vi "TDMS - File Viewer - KTMod1.vi"(4 "error in (no error)":errorcluster, 7 "file path":path) -> (0 "error out":errorcluster, 3 "file path out":path)   [LabVIEW 2019]
doc: "Developed by Kevin Thompson\nkevin@thompsonengineering.net\n\nCopyright 2020\nThompson Engineering, LLC\n<B>Copyright:</B> (c) 2017 National Instruments. All rights reserved.\n\nOpens the .tdms file specified in the <B>file path</B> input and presents the file data in the TDMS File Viewer dialog box."
uses:
  Instance           1 26Saved   TDMS - File Viewer .vi
  <vilib>/Utility/tdmsutil.llb/fileViewerConfigData.ctl
  <vilib>/Utility/tdmsutil.llb/TDMSFileViewerLocalizedText.vi
  <vilib>/Utility/error.llb/DialogType.ctl
  <vilib>/event_ctls.llb/sizeaction.ctl
  <vilib>/event_ctls.llb/panelstate.ctl
panel:
  out "LastXScaleFormat":u8
  out "TotalCount":u64
  out "Temp Configuration":T1
  in  "LastTopLeftValue":u64
  out "Resize?":bool
  in  "Help":bool
  in  "Status":string
  in  "Quit":bool
  in  "Settings...":bool
  in  "Properties / Values / Graph":T2(tab)
  in  "Properties":i32(listbox)
  in  "Go To":bool
  in  "Scrollbar":u64(c297)
  in  "Raw data values":i32(listbox)
  out "Waveform Graph":waveform(dbl)[](graph)
  in  "File contents":string(tree)
  # "Right Click for File Dialog"
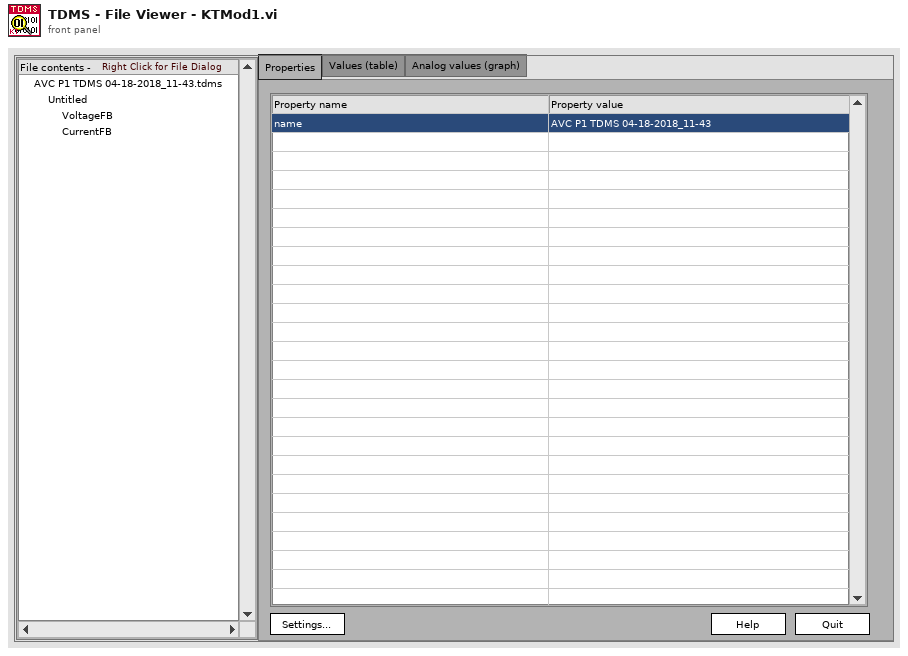
[diagram p1: front panel]
types:
  T1 = typedef "fileViewerConfigData.ctl" = cluster{"Show all (table)":bool, "Show all (graph)":bool, "limit (table)":u64, "limit (graph)":u64, "no show":bool, "start (table)":u64, "start (graph)":u64}
  T2 = enum32{"Properties", "Values (table)", "Analog values (graph)"}
  T3 = enum16{"open", "open or create", "create or replace", "create", "open (read-only)"}
  T4 = cluster{"Tree":refnum<vi>, "Tab Control":refnum<vi>, "property list":refnum<vi>, "raw data list":refnum<vi>, "Waveform Graph":refnum<vi>, "Ok":refnum<vi>, "Ok 2":refnum<vi>, "Ok 3":refnum<vi>, "Ok 4":refnum<vi>, "Scrollbar":refnum<vi>, "Ok 5":refnum<vi>, "TopLeftValue":refnum<vi>, "TotalCount":refnum<vi>}
  T5 = typedef "panelstate.ctl" = enum32{"Standard", "Minimized", "Maximized"}
  T6 = typedef "sizeaction.ctl" = enum32{"Minimized", "Maximized", "Resized"}
  T7 = cluster{"Shift":bool, "Ctrl":bool, "Alt":bool, "Cmd":bool, "Opt":bool}
  T8 = typedef "LVRectTypeDef.ctl" = cluster{"Left":i16, "Top":i16, "Right":i16, "Bottom":i16}
  T9 = typedef "LVRowAndColumnUnsignedTypeDef.ctl" = cluster{"Row":u32, "Column":u32}
  T10 = typedef "DialogType.ctl" = u16
  T11 = typedef "eventvkey.ctl" = enum16{"ASCII", "Enter", "Return", "Shift", "Ctrl", "Alt", "Cmd", "Opt", "Caps", "NumLock", "Clear", "Break", "Up", "Down", "Left", "Right", "Insert", "Delete", "Home", "End", "PageUp", "PageDown", "Escape", "Help", "Pause", "ScrollLock", "F1", "F2", "F3", "F4", "F5", "F6", "F7", "F8", "F9", "F10", "F11", "F12", "F13", "F14", "F15", "F16", "F17", "F18", "F19", "F20", "F21", "F22", "F23", "F24", "Play", "VolumeUp", "VolumeDown", "Mute", "Two Byte Char"}
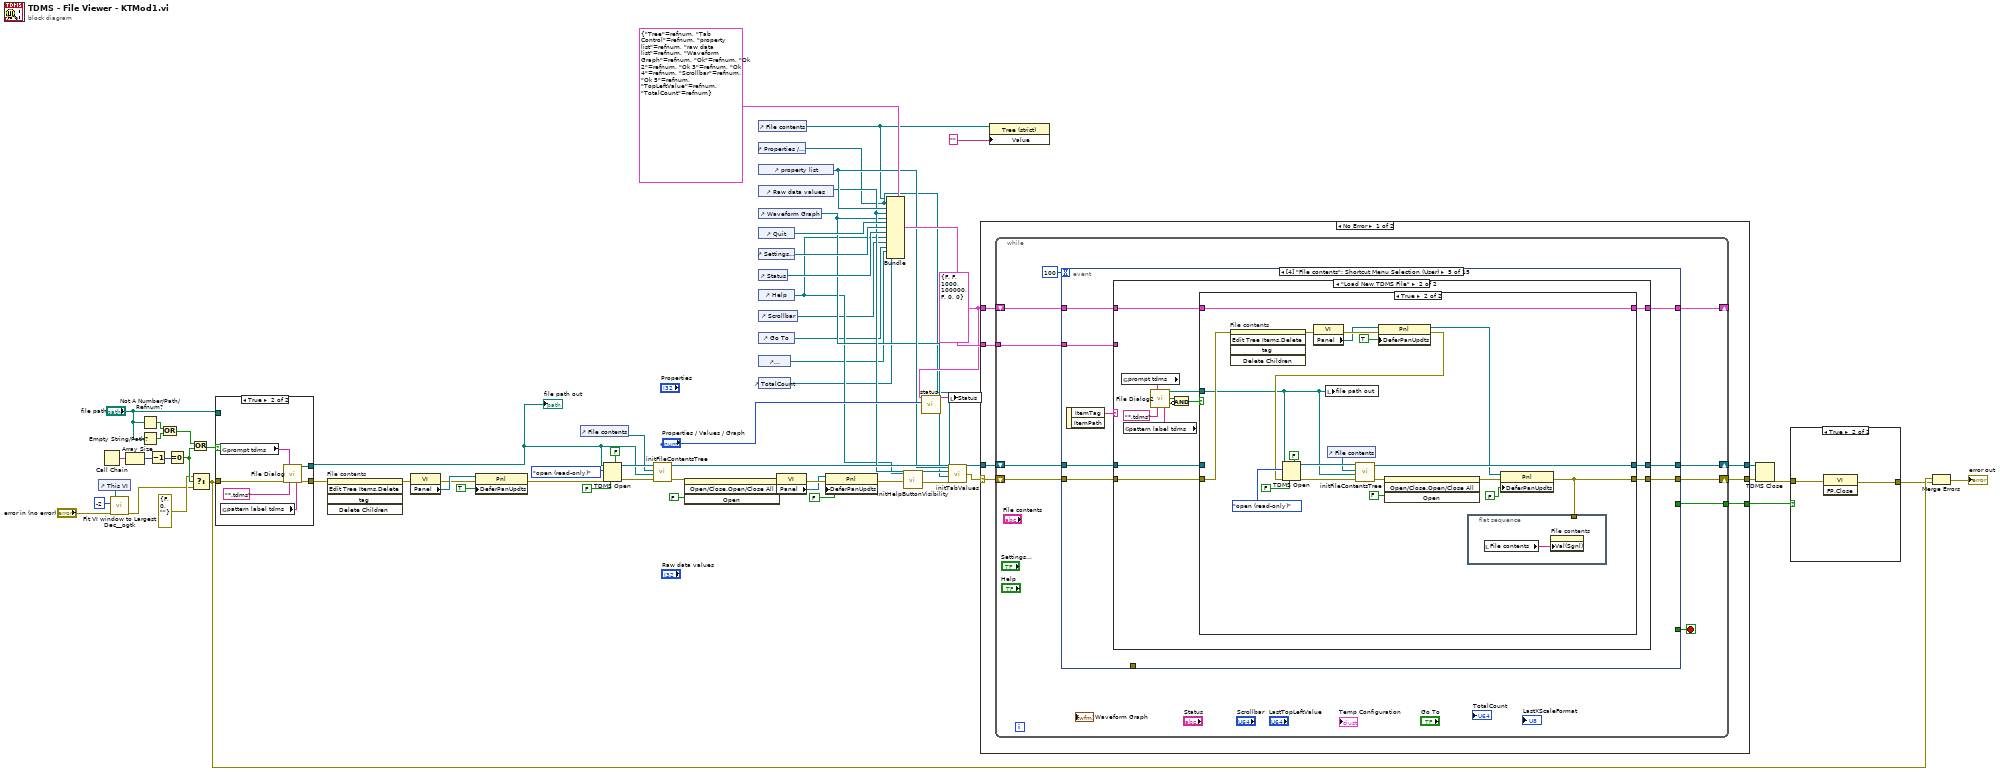
[diagram p0: block diagram]
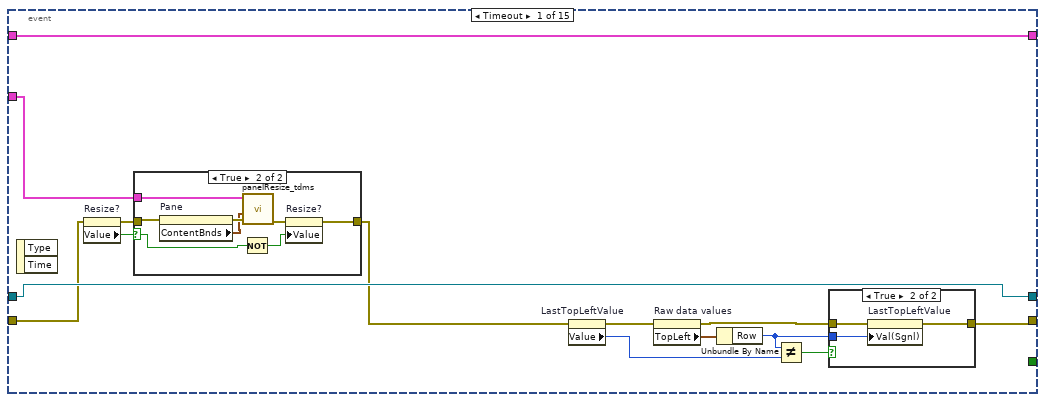
[diagram p3: hidden frame]
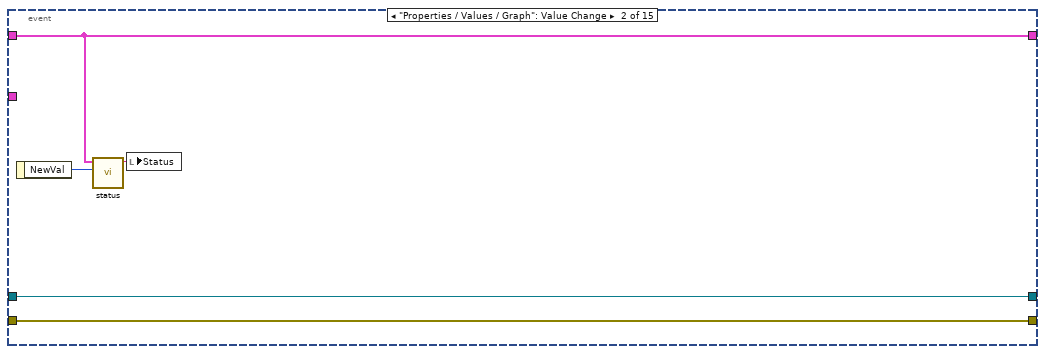
[diagram p6: hidden frame]
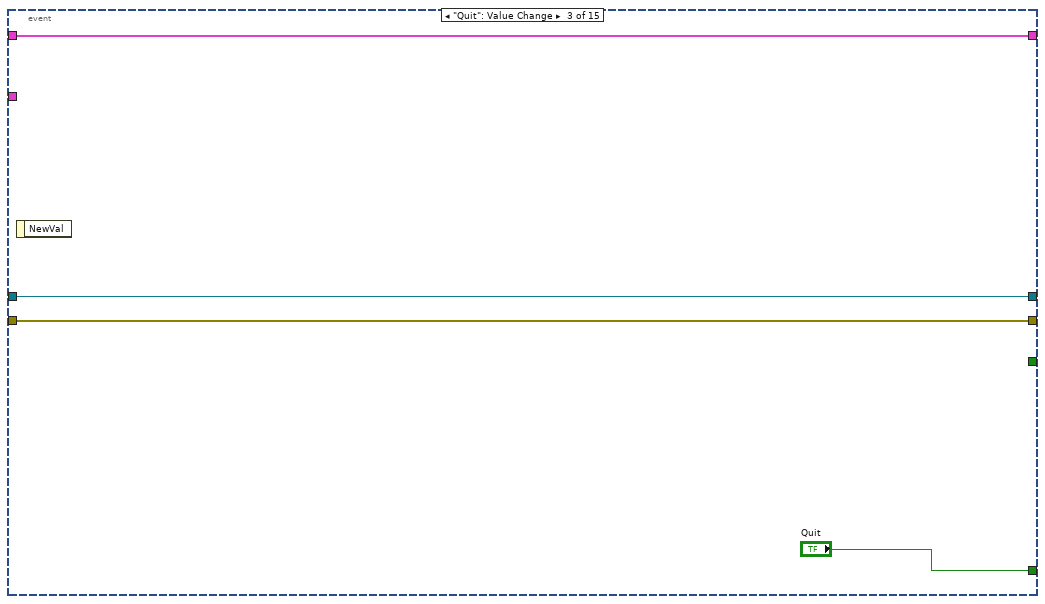
[diagram p7: hidden frame]
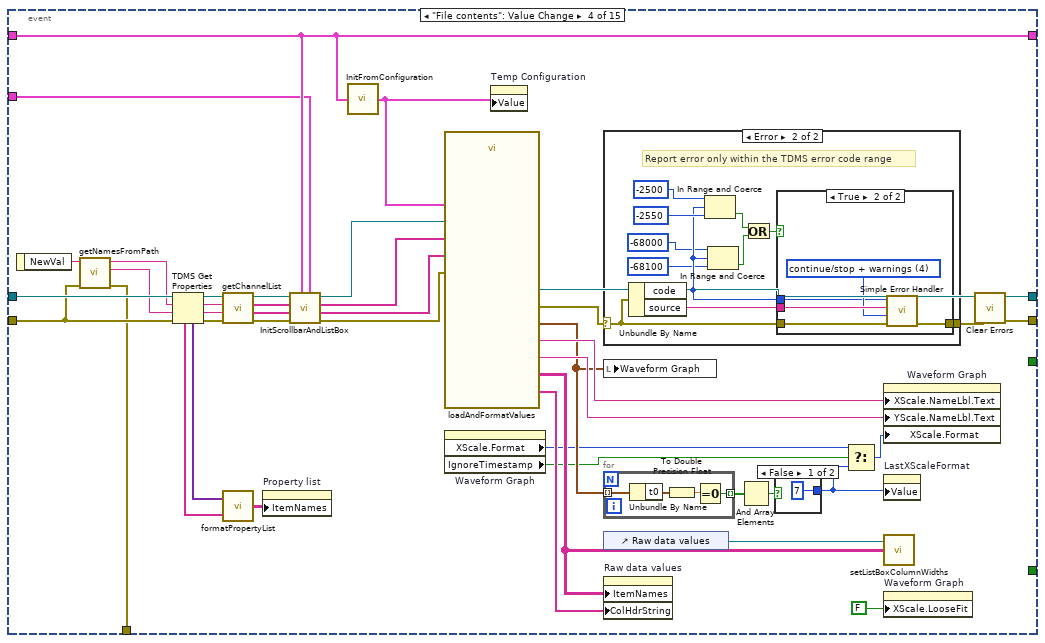
[diagram p8: hidden frame]
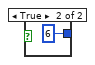
[diagram p9: hidden frame]
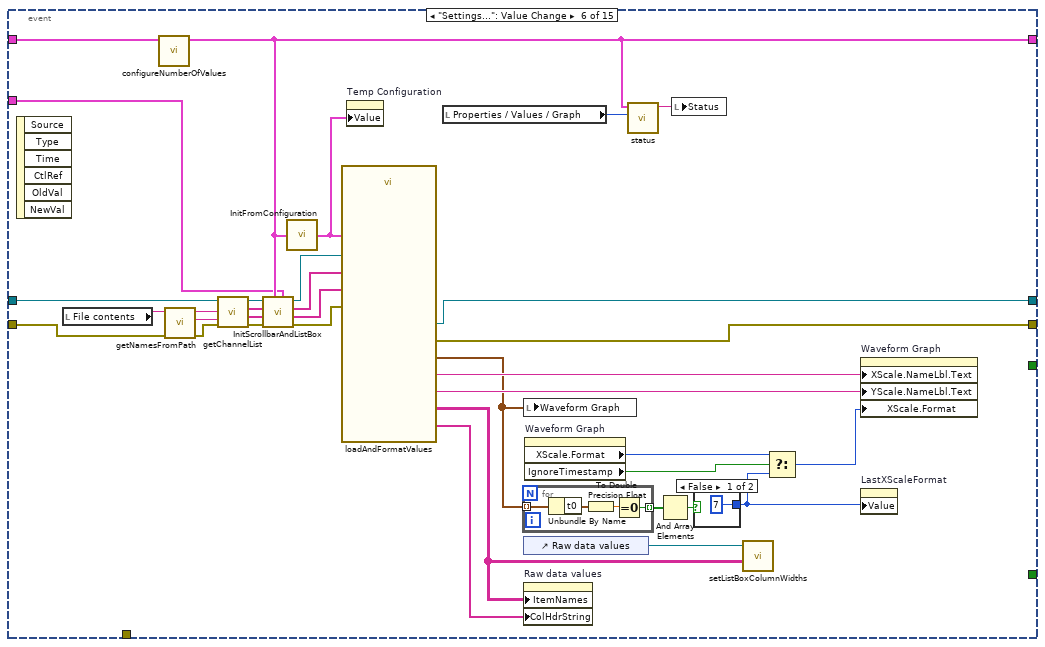
[diagram p14: hidden frame]
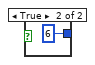
[diagram p15: hidden frame]
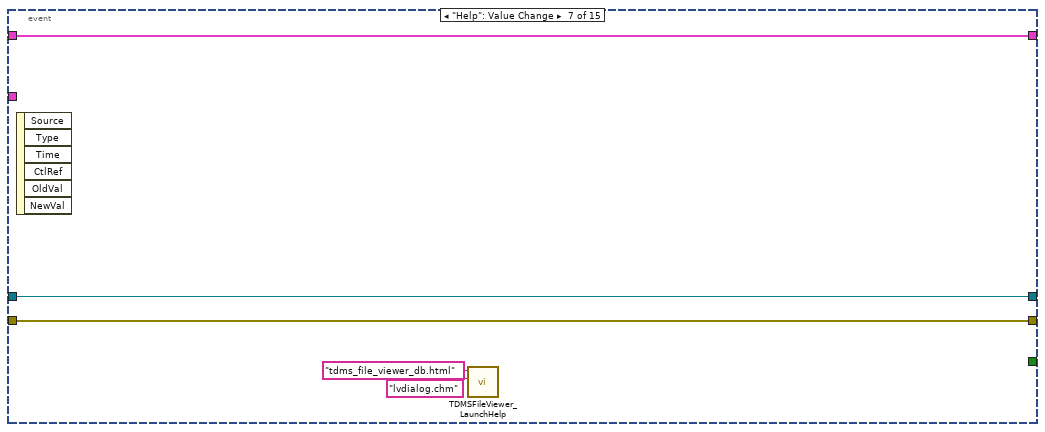
[diagram p16: hidden frame]
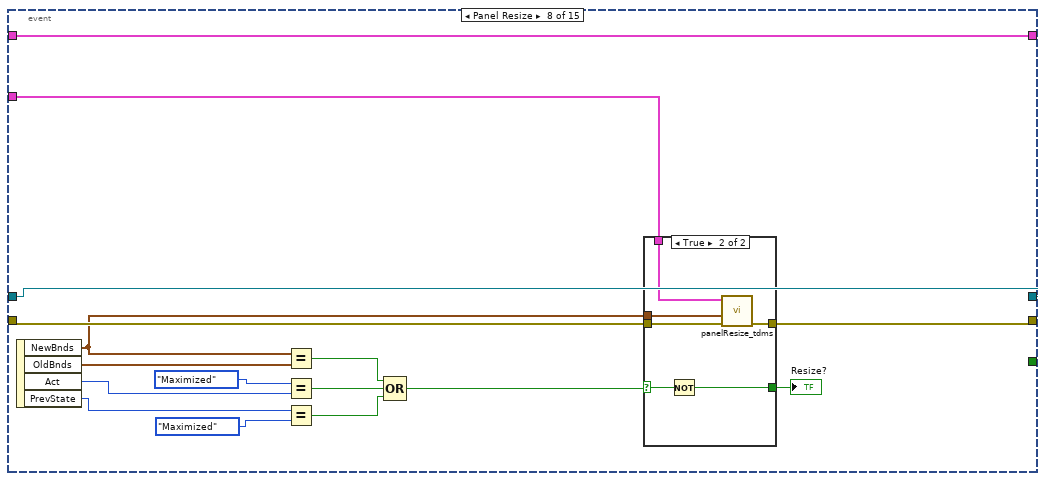
[diagram p17: hidden frame]
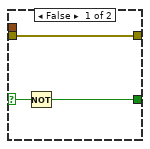
[diagram p18: hidden frame]
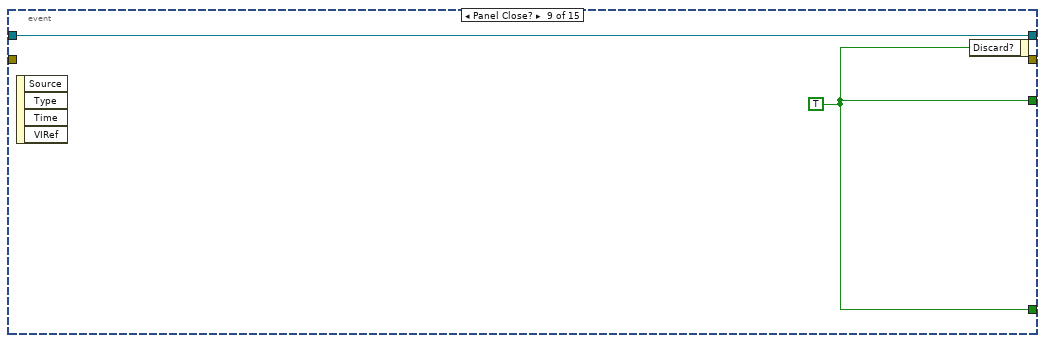
[diagram p19: hidden frame]
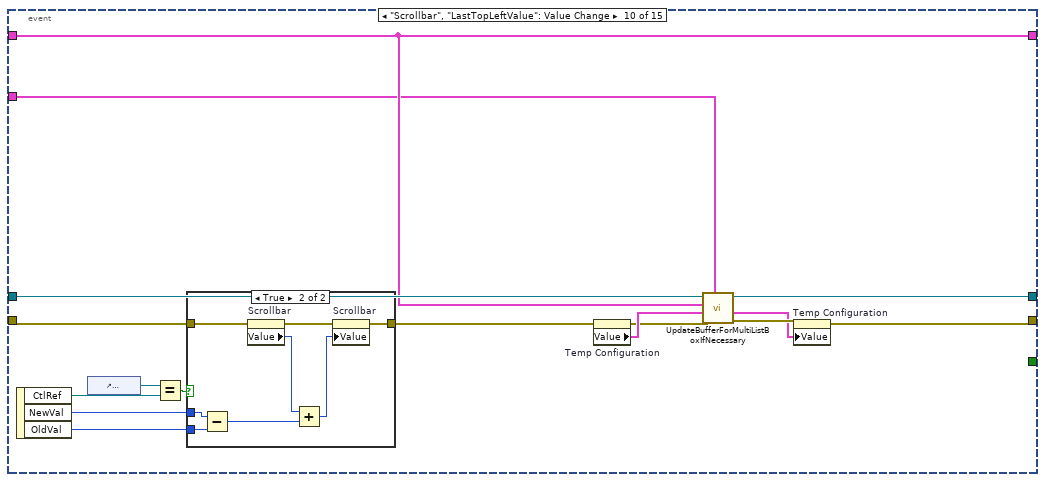
[diagram p20: hidden frame]
diagram:
  w29 = T1 {"Show all (table)"=FALSE, "Show all (graph)"=FALSE, "limit (table)"=1000, "limit (graph)"=100000, "no show"=FALSE, "start (table)"=0, "start (graph)"=0} ("TDMS File Viewer Configuration")
  n1 = control-ref of="This VI"() -> (w4:refnum<vi>)
  n2 = Call Chain() -> (call chain=w44:string[])
  n3 = call <userlib>:"Fit VI window to Largest Dec__ogtk.vi"("error in (no error)"="error in (no error)", "border spacing (2 px)"=-2, "VI Ref (calling VI)"=w4) -> ("error out"=w1:errorcluster)  [unwired: 3 in, 1 out]
  n4 = Array Size(array=w44) -> (size(s)=w42:i32)
  n5 = Not A Number/Path/Refnum?(number/path/refnum="file path") -> (NaN/Path/Refnum?=w46:bool)
  n6 = Empty String/Path?(string/path="file path") -> (empty?=w45:bool)
  n7 = Decrement(x=w42) -> (x-1=w41:i32)
  n8 = Or(x=w46, y=w45) -> (x .or. y?=w43:bool)
  n9 = Equal To 0?(x=w41) -> (x = 0?=w27:bool)
  n10 = Or(x=w43, y=w27) -> (x .or. y?=w40:bool)
  n11 = Select(t=errorcluster {"status"=FALSE, "code"=0, "source"=""}, s=w27, f=w1) -> (s? t:f=w11:errorcluster)
  n12 = case shown="True" w40 {
    tunnel: [w65 w71] -> w33
    tunnel: "file path" -> [w65 _]
    tunnel: [w64 w69] -> w32
    tunnel: w11 -> [w64 w68]
    frame False {
    }
    frame True {
      n13 = global read "TDMSFileViewerLocalizedText.vi" "prompt tdms"() -> (w67:string)
      n14 = global read "TDMSFileViewerLocalizedText.vi" "pattern label tdms"() -> (w66:string)
      n15 = call "File Dialog"("prompt"=w67, "error in"=w68, "pattern (all files)"="*.tdms", "pattern label"=w66) -> ("selected path"=w71:path, "error out"=w69:errorcluster)  [unwired: 3 in, 7 out]
    }
  }
  "file path out" <- w33
  n16 = invoke on="File contents" class="Tree (strict)" method="Edit Tree Items.Delete"(error in=w32) -> (error out=w54:errorcluster)  [unwired: 4 in, 4 out]
  n17 = property class="VI"(error in=w54) -> (error out=w55:errorcluster, "Panel"=w56:refnum<vi>)  [unwired: 1 in, 1 out]
  n18 = property class="Pnl"(reference=w56, error in=w55, "DeferPanUpdts"=TRUE ("Defer Panel Updates")) -> (error out=w58:errorcluster)  [unwired: 1 out]
  n19 = control-ref of="File contents"() -> (w34:refnum<vi>)
  n20 = TDMS Open(5:FALSE ("create index file? (T)"), 6:FALSE ("disable buffering (T)"), 8:w58, 10:T3."open (read-only)" ("operation"), 11:w33) -> (0:w63:errorcluster, 3:w62:refnum<k34>)  [unwired: 2 in]
  n21 = call <vilib>:"initFileContentsTree.vi"("error in (no error)"=w63, "file path"=w33, "Tree Refnum"=w34, "tdms file"=w62) -> ("error out"=w50:errorcluster, "tdms file out"=w61:refnum<k34>)  [unwired: 2 out]
  n22 = invoke on="File contents" class="Tree (strict)" method="Open/Close.Open/Close All"(error in=w50, "Open"=FALSE ("Open?")) -> (error out=w49:errorcluster)  [unwired: 2 in, 3 out]
  n23 = control-ref of="File contents"() -> (w17:refnum<vi>)
  n24 = control-ref of="property list"() -> (w21:refnum<vi>)
  n25 = control-ref of="Raw data values"() -> (w20:refnum<vi>)
  n26 = control-ref of="Waveform Graph"() -> (w19:refnum<vi>)
  n27 = control-ref of="Quit"() -> (w38:refnum<vi>)
  n28 = control-ref of="Settings..."() -> (w36:refnum<vi>)
  n29 = control-ref of="Status"() -> (w31:refnum<vi>)
  n30 = control-ref of="Help"() -> (w13:refnum<vi>)
  n31 = control-ref of="Scrollbar"() -> (w10:refnum<vi>)
  n32 = control-ref of="Go To"() -> (w9:refnum<vi>)
  n33 = control-ref of="LastTopLeftValue"() -> (w8:refnum<vi>)
  n34 = control-ref of="TotalCount"() -> (w7:refnum<vi>)
  n35 = control-ref of="Properties / Values / Graph"() -> (w18:refnum<vi>)
  n36 = property class="VI"(error in=w49) -> (error out=w52:errorcluster, "Panel"=w51:refnum<vi>)  [unwired: 1 in, 1 out]
  n37 = property class="Pnl"(reference=w51, error in=w52, "DeferPanUpdts"=FALSE ("Defer Panel Updates")) -> (error out=w15:errorcluster)  [unwired: 1 out]
  n38 = Bundle(cluster=T4 {"Tree"=refnum, "Tab Control"=refnum, "property list"=refnum, "raw data list"=refnum, "Waveform Graph"=refnum, "Ok"=refnum, "Ok 2"=refnum, "Ok 3"=refnum, "Ok 4"=refnum, "Scrollbar"=refnum, "Ok 5"=refnum, "TopLeftValue"=refnum, "TotalCount"=refnum} ("control refs"), "Tree"=w17, "Tab Control"=w18, "property list"=w21, "raw data list"=w20, "Waveform Graph"=w19, "Ok"=w38, "Ok 2"=w36, "Ok 3"=w31, "Ok 4"=w13, "Scrollbar"=w10, "Ok 5"=w9, "TopLeftValue"=w8, "TotalCount"=w7) -> (w39:T4)
  n39 = call <vilib>:"initHelpButtonVisibility.vi"("error in"=w15, "Help"=w13) -> ("error out"=w14:errorcluster)  [unwired: 9 in]
  n40 = call <vilib>:"status.vi"("tab sheet"="Properties / Values / Graph", "TDMS File Viewer Configuration"=w29) -> ("status"=w30:string)  [unwired: 5 out]
  n41 = local write "Status"(w30) -> ()
  n42 = call <vilib>:"initTabValues.vi"("properties"=w21, "Values"=w20, "waveform"=w19, "error in"=w14, "Properties / Values / Graph"=w18) -> ("error out"=w22:errorcluster)
  n43 = case shown="No Error" w22 {
    selector: w22 -> [w73 w444]
    tunnel: w61 -> [w78 w445]
    tunnel: [w77 w445] -> w60
    tunnel: [w76 w443] -> w59
    tunnel: w39 -> [w75 _]
    tunnel: w29 -> [w74 _]
    tunnel: [w72 FALSE] -> w25
    frame No Error {
      n44 = while {
        shift-right: [w86] -> w76
        shift-left: w73 -> [w87]
        shift-right: [w85] -> w77
        shift-left: w78 -> [w88]
        tunnel: w75 -> [w83]
        shift-right: [w81] -> _
        shift-left: w74 -> [w82]
        tunnel: [w80] -> w72
        stop <- w84 stop-if-true
        n45 = event shown="[4] \"File contents\": Shortcut Menu Selection (User)" {
          selector: _ -> [_ _ _ _ _ _ _ _ _ _ _ _ _ _ _]
          dyn-events: _ -> [_ _ _ _ _ _ _ _ _ _ _ _ _ _ _]
          timeout: 100 -> [_ _ _ _ _ _ _ _ _ _ _ _ _ _ _]
          tunnel: w88 -> [w102 w119 w123 w165 w193 w262 w282 w299 w310 w326 w345 w370 w385 w418 w435]
          tunnel: w87 -> [w97 w120 w122 w157 w191 w269 w281 w297 _ w313 w337 w359 w382 w417 w434]
          tunnel: [w90 w120 w122 w153 w190 w270 w281 w296 _ w320 w342 w362 w383 w417 w426] -> w86
          tunnel: [w102 w119 w123 w164 w192 w271 w282 w299 w310 w325 w344 w369 w384 w418 w435] -> w85
          tunnel: [_ _ "Quit" _ _ _ _ _ w309 _ _ _ _ _ _] -> w84
          tunnel: [_ _ _ w156 _ _ _ _ _ _ _ _ _ _ _] -> _
          tunnel: w83 -> [w98 _ _ w132 w196 w246 _ w298 _ w312 w338 w360 w379 _ _]
          tunnel: w82 -> [w101 w116 w121 w133 w195 w272 w283 w295 _ w324 w346 w371 w386 w419 w436]
          tunnel: [w101 w116 w121 w133 w194 w248 w283 w295 _ w324 w346 w371 w386 w419 w436] -> w81
          tunnel: [_ _ _ _ _ _ _ _ w309 _ _ _ _ _ _] -> w80
          event Timeout {
            n46 = event-data() -> ()  [unwired: 3 out]
            n47 = property on="Resize?" class="Bool (strict)"(error in=w97) -> (error out=w99:errorcluster, "Value"=w100:bool)  [unwired: 1 in, 1 out]
            n48 = case shown="True" w100 {
              selector: w100 -> [_ w114]
              tunnel: w98 -> [_ w115]
              tunnel: w99 -> [w107 w110]
              tunnel: [w107 w112] -> w95
              frame False {
              }
              frame True {
                n49 = property on="Pane" class="Pane"(error in=w110) -> (error out=w109:errorcluster, "ContentBnds"=w108:T8)  [unwired: 1 in, 1 out]
                n50 = Not(x=w114) -> (.not. x?=w111:bool)
                n51 = call <vilib>:"panelResize_tdms.vi"("error in (no error)"=w109, "NewBnds"=w108, "control refs"=w115) -> ("error out"=w113:errorcluster)  [unwired: 4 in]
                n52 = property on="Resize?" class="Bool (strict)"(error in=w113, "Value"=w111) -> (error out=w112:errorcluster)  [unwired: 1 in, 1 out]
              }
            }
            n53 = property on="LastTopLeftValue" class="DigNum (strict)"(error in=w95) -> (error out=w94:errorcluster, "Value"=w93:u64)  [unwired: 1 in, 1 out]
            n54 = property on="Raw data values" class="MCListbox (strict)"(error in=w94) -> (error out=w91:errorcluster, "TopLeft"=w96:T9)  [unwired: 1 in, 1 out]
            n55 = Unbundle By Name(w96) -> ("Row"=w89:u32)
            n56 = Not Equal?(x=w89, y=w93) -> (x != y?=w92:bool)
            n57 = case shown="True" w92 {
              tunnel: w91 -> [w103 w106]
              tunnel: [w103 w105] -> w90
              tunnel: w89 -> [_ w104]
              frame False {
              }
              frame True {
                n58 = property on="LastTopLeftValue" class="DigNum (strict)"(error in=w106, "Val(Sgnl)"=w104) -> (error out=w105:errorcluster)  [unwired: 1 in, 1 out]
              }
            }
          }
          event "Properties / Values / Graph": Value Change {
            n59 = event-data() -> ("NewVal"=w118:T2)  [unwired: 1 out]
            n60 = call <vilib>:"status.vi"("tab sheet"=w118, "TDMS File Viewer Configuration"=w116) -> ("status"=w117:string)  [unwired: 5 out]
            n61 = local write "Status"(w117) -> ()
          }
          event "Quit": Value Change {
            n62 = event-data() -> ()  [unwired: 2 out]
          }
          event "File contents": Value Change {
            n63 = event-data() -> ("NewVal"=w159:string)  [unwired: 1 out]
            n64 = call <vilib>:"getNamesFromPath.vi"("error in (no error)"=w157, "tree path"=w159) -> ("error out"=w156:errorcluster, "channel"=w162:string, "group"=w163:string)  [unwired: 3 out]
            n65 = TDMS Get Properties(8:w157, 9:w162, 10:w163, 11:w165) -> (0:w151:errorcluster, 1:w150:string, 2:w146:string, 3:w152:refnum<k34>, 4:w160:variant[], 6:w161:string[])  [unwired: 2 out]
            n66 = call <vilib>:"getChannelList.vi"("error in (no error)"=w151, "channel names"=w150, "group name"=w146, "tdms file"=w152) -> ("error out"=w141:errorcluster, "channel names out"=w139:string[], "group names out"=w137:string[], "tdms file out"=w135:refnum<k34>)
            n67 = call <vilib>:"formatPropertyList.vi"("property names"=w161, "property values"=w160) -> ("strings"=w158:string[][])
            n68 = property on="Property list" class="MCListbox (strict)"("ItemNames"=w158) -> ()  [unwired: 2 in, 2 out]
            n69 = call <vilib>:"InitScrollbarAndListBox.vi"("control refs"=w132, "configuration"=w133, "error in (no error)"=w141, "channel names"=w139, "group names"=w137, "tdms in"=w135) -> ("error out"=w140:errorcluster, "channel out"=w138:string[], "group out"=w136:string[], "tdms out"=w134:refnum<k34>)  [unwired: 2 in]
            n70 = call <vilib>:"InitFromConfiguration.vi"("configuration"=w133) -> ("output cluster"=w142:T1)  [unwired: 4 in]
            n71 = call <vilib>:"loadAndFormatValues.vi"("error in (no error)"=w140, "configuration"=w142, "channel names"=w138, "group names"=w136, "tdms file"=w134) -> ("error out"=w145:errorcluster, "graph y names"=w148:string, "graph x names"=w147:string, "tdms file out"=w164:refnum<k34>, "waveform values"=w131:waveform(dbl)[], "table values"=w155:string[][], "table headers"=w149:string[])
            n72 = property on="Waveform Graph" class="WFGraph (strict)"() -> ("XScale.Format"=w126:u8, "IgnoreTimestamp"=w125:bool)  [unwired: 2 in, 2 out]
            n73 = property on="Temp Configuration" class="Clust (strict)"("Value"=w142) -> ()  [unwired: 2 in, 2 out]
            n74 = case shown="Error" w145 {
              selector: w145 -> [w172 w182]
              tunnel: [w172 w181] -> w144
              frame No Error {
              }
              frame Error {
                # "Report error only within the TDMS error code range"
                n75 = Unbundle By Name(w182) -> ("code"=w178:i32, "source"=w183:string)
                n76 = In Range and Coerce(upper limit=-2500, x=w178, lower limit=-2550 ("upper limit")) -> (In Range?=w175:bool)  [unwired: 1 out]
                n77 = In Range and Coerce(upper limit=-68000, x=w178, lower limit=-68100) -> (In Range?=w174:bool)  [unwired: 1 out]
                n78 = Or(x=w175, y=w174) -> (x .or. y?=w173:bool)
                n79 = case shown="True" w173 {
                  tunnel: w183 -> [_ w189]
                  tunnel: w182 -> [w184 w188]
                  tunnel: [w184 w187] -> w181
                  tunnel: w178 -> [_ w185]
                  frame False {
                    # "Out of the range of TDMS\nerror code, we don't report\nthem."
                  }
                  frame True {
                    w186 = T10 4 items=["no dialog", "OK message", "continue or stop message", "OK message + warnings", "continue/stop + warnings"] ("type of dialog (OK msg:1)")
                    n80 = call <vilib>:"Simple Error Handler.vi"("error code (no error:0)"=w185, "error source (\" \")"=w189, "type of dialog (OK msg:1)"=w186, "error in (no error)"=w188) -> ("error out"=w187:errorcluster)  [unwired: 1 in, 4 out]
                  }
                }
              }
            }
            n81 = local write "Waveform Graph"(w131) -> ()
            n82 = for {
              tunnel: w131 -> [w171] mode=indexing
              tunnel: [w168] -> w130 mode=indexing
              n83 = Unbundle By Name(w171) -> ("t0"=w170:timestamp)
              n84 = To Double Precision Float(number=w170) -> (double precision float=w169:dbl)
              n85 = Equal To 0?(x=w169) -> (x = 0?=w168:bool)
            }
            n86 = control-ref of="Raw data values"() -> (w154:refnum<vi>)
            n87 = property on="Raw data values" class="MCListbox (strict)"("ItemNames"=w155, "ColHdrString"=w149) -> ()  [unwired: 2 in, 2 out]
            n88 = And Array Elements(Boolean array=w130) -> (logical AND=w129:bool)
            n89 = case shown="False" w129 {
              tunnel: [u8 7 u8 6] -> w127
              frame False {
              }
              frame True {
              }
            }
            n90 = Select(t=w126, s=w125, f=w127) -> (s? t:f=w128:u8)
            n91 = property on="Waveform Graph" class="WFGraph (strict)"("XScale.NameLbl.Text"=w147, "YScale.NameLbl.Text"=w148, "XScale.Format"=w128) -> ()  [unwired: 2 in, 2 out]
            n92 = property on="LastXScaleFormat" class="DigNum (strict)"("Value"=w127) -> ()  [unwired: 2 in, 2 out]
            n93 = call <vilib>:"setListBoxColumnWidths.vi"("table data"=w155, "MCListbox Refnum"=w154) -> ()  [unwired: 1 out]
            n94 = property on="Waveform Graph" class="WFGraph (strict)"("XScale.LooseFit"=FALSE ("X Scale.Loose Fit")) -> ()  [unwired: 2 in, 2 out]
            n95 = call <vilib>:"Clear Errors.vi"("error in (no error)"=w144) -> ("error out"=w153:errorcluster)  [unwired: 1 in, 5 out]
          }
          event "File contents": Shortcut Menu Selection (User) {
            n96 = event-data() -> ("ItemTag"=w197:string)  [unwired: 2 out]
            n97 = case shown="\"Load New TDMS File\"" w197 {
              tunnel: w196 -> [_ _]
              tunnel: w195 -> [w200 w207]
              tunnel: [w200 w206] -> w194
              tunnel: w193 -> [w199 w205]
              tunnel: [w199 w203] -> w192
              tunnel: w191 -> [w198 w204]
              tunnel: [w198 w202] -> w190
              frame "False", Default {
              }
              frame "Load New TDMS File" {
                n98 = global read "TDMSFileViewerLocalizedText.vi" "prompt tdms"() -> (w212:string)
                n99 = global read "TDMSFileViewerLocalizedText.vi" "pattern label tdms"() -> (w213:string)
                n100 = call "File Dialog2"("prompt"=w212, "pattern (all files)"="*.tdms", "pattern label"=w213) -> ("selected path"=w201:path, "exists"=w210:bool, "cancelled"=w209:bool)  [unwired: 4 in, 6 out]
                n101 = Compound Arithmetic op=AND(w210, invert w209) -> (w208:bool)
                n102 = case shown="True" w208 {
                  tunnel: [w216 w237] -> w206
                  tunnel: w207 -> [w216 w237]
                  tunnel: w205 -> [w215 _]
                  tunnel: w204 -> [w214 w236]
                  tunnel: [w215 w220] -> w203
                  tunnel: [w214 w217] -> w202
                  tunnel: w201 -> [_ w225]
                  frame False {
                  }
                  frame True {
                    n103 = invoke on="File contents" class="Tree (strict)" method="Edit Tree Items.Delete"(error in=w236) -> (error out=w232:errorcluster)  [unwired: 4 in, 4 out]
                    n104 = property class="VI"(error in=w232) -> (error out=w235:errorcluster, "Panel"=w234:refnum<vi>)  [unwired: 1 in, 1 out]
                    n105 = local write "file path out"(w225) -> ()
                    n106 = control-ref of="File contents"() -> (w224:refnum<vi>)
                    n107 = property class="Pnl"(reference=w234, error in=w235, "DeferPanUpdts"=TRUE ("Defer Panel Updates")) -> (reference out=w219:refnum<vi>, error out=w228:errorcluster)
                    n108 = TDMS Open(5:FALSE ("create index file? (T)"), 6:FALSE ("disable buffering (T)"), 8:w228, 10:T3."open (read-only)" ("operation"), 11:w225) -> (0:w227:errorcluster, 3:w226:refnum<k34>)  [unwired: 2 in]
                    n109 = call <vilib>:"initFileContentsTree.vi"("error in (no error)"=w227, "file path"=w225, "Tree Refnum"=w224, "tdms file"=w226) -> ("error out"=w222:errorcluster, "tdms file out"=w220:refnum<k34>)  [unwired: 2 out]
                    n110 = invoke on="File contents" class="Tree (strict)" method="Open/Close.Open/Close All"(error in=w222, "Open"=FALSE ("Open?")) -> (error out=w218:errorcluster)  [unwired: 2 in, 3 out]
                    n111 = flat-sequence {
                      tunnel: w217 -> [_]
                      frame #0 {
                        n112 = local read "File contents"() -> (w238:string)
                        n113 = property on="File contents" class="Tree (strict)"("Val(Sgnl)"=w238) -> ()  [unwired: 2 in, 2 out]
                      }
                    }
                    n114 = property class="Pnl"(reference=w219, error in=w218, "DeferPanUpdts"=FALSE ("Defer Panel Updates")) -> (error out=w217:errorcluster)  [unwired: 1 out]
                  }
                }
              }
            }
          }
          event "Settings...": Value Change {
            n115 = event-data() -> ()  [unwired: 7 out]
            n116 = local read "File contents"() -> (w263:string)
            n117 = call <vilib>:"configureNumberOfValues.vi"("TDMS File Viewer Configuration"=w272) -> ("TDMS File Viewer Configuration Out"=w248:T1)  [unwired: 10 out]
            n118 = call <vilib>:"getNamesFromPath.vi"("error in (no error)"=w269, "tree path"=w263) -> ("error out"=w261:errorcluster, "channel"=w259:string, "group"=w260:string)  [unwired: 3 out]
            n119 = call <vilib>:"getChannelList.vi"("error in (no error)"=w261, "channel names"=w259, "group name"=w260, "tdms file"=w262) -> ("error out"=w250:errorcluster, "channel names out"=w252:string[], "group names out"=w254:string[], "tdms file out"=w256:refnum<k34>)
            n120 = call <vilib>:"InitScrollbarAndListBox.vi"("control refs"=w246, "configuration"=w248, "error in (no error)"=w250, "channel names"=w252, "group names"=w254, "tdms in"=w256) -> ("error out"=w249:errorcluster, "channel out"=w251:string[], "group out"=w253:string[], "tdms out"=w255:refnum<k34>)  [unwired: 2 in]
            n121 = call <vilib>:"InitFromConfiguration.vi"("configuration"=w248) -> ("output cluster"=w247:T1)  [unwired: 4 in]
            n122 = call <vilib>:"loadAndFormatValues.vi"("error in (no error)"=w249, "configuration"=w247, "channel names"=w251, "group names"=w253, "tdms file"=w255) -> ("error out"=w270:errorcluster, "graph y names"=w265:string, "graph x names"=w264:string, "tdms file out"=w271:refnum<k34>, "waveform values"=w243:waveform(dbl)[], "table values"=w266:string[][], "table headers"=w268:string[])
            n123 = property on="Temp Configuration" class="Clust (strict)"("Value"=w247) -> ()  [unwired: 2 in, 2 out]
            n124 = local read "Properties / Values / Graph"() -> (w257:T2)
            n125 = for {
              tunnel: w243 -> [w278] mode=indexing
              tunnel: [w275] -> w245 mode=indexing
              n126 = Unbundle By Name(w278) -> ("t0"=w277:timestamp)
              n127 = To Double Precision Float(number=w277) -> (double precision float=w276:dbl)
              n128 = Equal To 0?(x=w276) -> (x = 0?=w275:bool)
            }
            n129 = local write "Waveform Graph"(w243) -> ()
            n130 = control-ref of="Raw data values"() -> (w267:refnum<vi>)
            n131 = property on="Raw data values" class="MCListbox (strict)"("ItemNames"=w266, "ColHdrString"=w268) -> ()  [unwired: 2 in, 2 out]
            n132 = property on="Waveform Graph" class="WFGraph (strict)"() -> ("XScale.Format"=w240:u8, "IgnoreTimestamp"=w239:bool)  [unwired: 2 in, 2 out]
            n133 = call <vilib>:"status.vi"("tab sheet"=w257, "TDMS File Viewer Configuration"=w248) -> ("status"=w258:string)  [unwired: 5 out]
            n134 = And Array Elements(Boolean array=w245) -> (logical AND=w244:bool)
            n135 = local write "Status"(w258) -> ()
            n136 = case shown="False" w244 {
              tunnel: [u8 7 u8 6] -> w241
              frame False {
              }
              frame True {
              }
            }
            n137 = call <vilib>:"setListBoxColumnWidths.vi"("table data"=w266, "MCListbox Refnum"=w267) -> ()  [unwired: 1 out]
            n138 = Select(t=w240, s=w239, f=w241) -> (s? t:f=w242:u8)
            n139 = property on="Waveform Graph" class="WFGraph (strict)"("XScale.NameLbl.Text"=w264, "YScale.NameLbl.Text"=w265, "XScale.Format"=w242) -> ()  [unwired: 2 in, 2 out]
            n140 = property on="LastXScaleFormat" class="DigNum (strict)"("Value"=w241) -> ()  [unwired: 2 in, 2 out]
          }
          event "Help": Value Change {
            n141 = event-data() -> ()  [unwired: 7 out]
            n142 = call <vilib>:"TDMSFileViewer_LaunchHelp.vi"("CHM or HLP filename (lvdialog.chm)"="lvdialog.chm", "HTML filename"="tdms_file_viewer_db.html") -> ()  [unwired: 1 in, 5 out]
          }
          event Panel Resize {
            n143 = event-data() -> ("NewBnds"=w287:T8, "OldBnds"=w286:T8, "Act"=w288:T6, "PrevState"=w289:T5)  [unwired: 1 out]
            n144 = Equal?(x=w287, y=w286) -> (x = y?=w292:bool)
            n145 = Equal?(x=sizeaction."Maximized" ("Act"), y=w288) -> (x = y?=w291:bool)
            n146 = Equal?(x=w289, y=panelstate."Maximized" ("PrevState")) -> (x = y?=w290:bool)
            n147 = Compound Arithmetic op=OR(w292, w291, w290) -> (w285:bool)
            n148 = case shown="True" w285 {
              selector: w285 -> [w301 w304]
              tunnel: w298 -> [_ w308]
              tunnel: w297 -> [w302 w307]
              tunnel: [w302 w306] -> w296
              tunnel: w287 -> [_ w305]
              tunnel: [w300 w303] -> w284
              frame False {
                n149 = Not(x=w301) -> (.not. x?=w300:bool)
              }
              frame True {
                n150 = Not(x=w304) -> (.not. x?=w303:bool)
                n151 = call <vilib>:"panelResize_tdms.vi"("error in (no error)"=w307, "NewBnds"=w305, "control refs"=w308) -> ("error out"=w306:errorcluster)  [unwired: 4 in]
              }
            }
            "Resize?" <- w284
          }
          event Panel Close? {
            w309 = TRUE
            n152 = event-data() -> ()  [unwired: 5 out]
            n153 = event-data("Discard?"=w309) -> ()  [unwired: 1 in, 1 out]
          }
          event "Scrollbar", "LastTopLeftValue": Value Change {
            n154 = event-data() -> ("CtlRef"=w318:refnum<vi>, "NewVal"=w315:u64, "OldVal"=w314:u64)  [unwired: 1 out]
            n155 = control-ref of="LastTopLeftValue"() -> (w317:refnum<vi>)
            n156 = Equal?(x=w317, y=w318) -> (x = y?=w316:bool)
            n157 = case shown="True" w316 {
              tunnel: w315 -> [_ w331]
              tunnel: w314 -> [_ w330]
              tunnel: w313 -> [w327 w329]
              tunnel: [w327 w328] -> w311
              frame False {
              }
              frame True {
                n158 = Subtract(x=w331, y=w330) -> (x-y=w333:u64)
                n159 = property on="Scrollbar" class="Scroll (strict)"(error in=w329) -> (error out=w335:errorcluster, "Value"=w334:u64)  [unwired: 1 in, 1 out]
                n160 = Add(x=w334, y=w333) -> (x+y=w332:u64)
                n161 = property on="Scrollbar" class="Scroll (strict)"(error in=w335, "Value"=w332) -> (error out=w328:errorcluster)  [unwired: 1 in, 1 out]
              }
            }
            n162 = property on="Temp Configuration" class="Clust (strict)"(error in=w311) -> (error out=w322:errorcluster, "Value"=w323:T1)  [unwired: 1 in, 1 out]
            n163 = call <vilib>:"UpdateBufferForMultiListBoxIfNecessary.vi"("control refs"=w312, "error in"=w322, "Buffer Configuration"=w323, "TDMS File Viewer Configuration"=w324, "tdms file in"=w326) -> ("error out"=w321:errorcluster, "BufferConfig out"=w319:T1, "tdms file out"=w325:refnum<k34>)  [unwired: 4 in]
            n164 = property on="Temp Configuration" class="Clust (strict)"(error in=w321, "Value"=w319) -> (error out=w320:errorcluster)  [unwired: 1 in, 1 out]
          }
          event "Raw data values": Key Down?; "Raw data values": event type 3.0.x8000000b {
            n165 = event-data() -> ("VKey"=w340:T11)  [unwired: 1 out]
            n166 = call <vilib>:"UpdateScrollbarBeforeKeyEvent.vi"("error in (no error)"=w337, "VKey"=w340, "control refs 2"=w338) -> ("error out"=w343:errorcluster, "LoadBuffer?"=w341:bool, "DiscardEvent?"=w339:bool)  [unwired: 6 in]
            n167 = case shown="True" w341 {
              tunnel: w346 -> [_ w354]
              tunnel: w345 -> [w347 w353]
              tunnel: [w347 w352] -> w344
              tunnel: w343 -> [w348 w349]
              tunnel: [w348 w351] -> w336
              tunnel: w338 -> [_ w350]
              frame False {
              }
              frame True {
                n168 = property on="Temp Configuration" class="Clust (strict)"(error in=w349) -> (error out=w357:errorcluster, "Value"=w358:T1)  [unwired: 1 in, 1 out]
                n169 = call <vilib>:"UpdateBufferForMultiListBoxIfNecessary.vi"("control refs"=w350, "error in"=w357, "Buffer Configuration"=w358, "TDMS File Viewer Configuration"=w354, "tdms file in"=w353) -> ("error out"=w356:errorcluster, "BufferConfig out"=w355:T1, "tdms file out"=w352:refnum<k34>)  [unwired: 4 in]
                n170 = property on="Temp Configuration" class="Clust (strict)"(error in=w356, "Value"=w355) -> (error out=w351:errorcluster)  [unwired: 1 in, 1 out]
              }
            }
            n171 = call <vilib>:"UpdateListBoxAfterKeyEvent.vi"("DiscardEvent?"=w339, "error in (no error)"=w336, "VKey"=w340, "control refs"=w338) -> ("error out"=w342:errorcluster)  [unwired: 7 in]
            n172 = event-data("Discard?"=w339) -> ()  [unwired: 1 in, 1 out]
          }
          event "Go To": Value Change {
            n173 = event-data() -> ()  [unwired: 2 out]
            n174 = call <vilib>:"GoTo.vi"("error in"=w359, "control refs"=w360) -> ("error out"=w368:errorcluster, "VisibleValue"=w365:u64)  [unwired: 8 in]
            n175 = property on="Temp Configuration" class="Clust (strict)"(error in=w368) -> (error out=w374:errorcluster, "Value"=w375:T1)  [unwired: 1 in, 1 out]
            n176 = call <vilib>:"UpdateBufferForMultiListBoxIfNecessary.vi"("control refs"=w360, "error in"=w374, "Buffer Configuration"=w375, "TDMS File Viewer Configuration"=w371, "tdms file in"=w370) -> ("error out"=w373:errorcluster, "BufferConfig out"=w372:T1, "tdms file out"=w369:refnum<k34>)  [unwired: 4 in]
            n177 = property on="Temp Configuration" class="Clust (strict)"(error in=w373, "Value"=w372) -> (error out=w361:errorcluster)  [unwired: 1 in, 1 out]
            n178 = property on="Raw data values" class="MCListbox (strict)"(error in=w361) -> (error out=w363:errorcluster, "TopLeft"=w367:T9)  [unwired: 1 in, 1 out]
            n179 = Unbundle By Name(w367) -> ("Row"=w366:u32)
            n180 = Add(x=w366, y=w365) -> (x+y=w364:u64)
            n181 = property on="Raw data values" class="MCListbox (strict)"(error in=w363, "Value"=w364) -> (error out=w362:errorcluster)  [unwired: 1 in, 1 out]
          }
          event Key Down {
            n182 = event-data() -> ("PlatMods"=w378:T7, "Char"=w377:i16)  [unwired: 1 out]
            n183 = property on="Raw data values" class="MCListbox (strict)"(error in=w382) -> (error out=w376:errorcluster, "Key Focus"=w381:bool)  [unwired: 1 in, 1 out]
            n184 = case shown="True" w381 {
              selector: w381 -> [w387 _]
              tunnel: [w387 w388] -> w380
              tunnel: w378 -> [_ w393]
              tunnel: w377 -> [_ w392]
              frame False {
              }
              frame True {
                n185 = disable-structure shown="Default" {
                  disable-tunnel: [T7 {"Shift"=FALSE, "Ctrl"=TRUE, "Alt"=FALSE, "Cmd"=FALSE, "Opt"=TRUE} ("PlatMods") T7 {"Shift"=FALSE, "Ctrl"=FALSE, "Alt"=FALSE, "Cmd"=TRUE, "Opt"=FALSE} ("PlatMods")] -> w394
                  frame condition #0 (active) {
                  }
                  frame condition #1 {
                  }
                }
                n186 = Equal?(x=w394, y=w393) -> (x = y?=w390:bool)
                n187 = Equal?(x=w392, y=i16 103 ("Char")) -> (x = y?=w389:bool)
                n188 = And(x=w390, y=w389) -> (x .and. y?=w388:bool)
              }
            }
            n189 = case shown="True" w380 {
              tunnel: w386 -> [_ w412]
              tunnel: w385 -> [w397 w411]
              tunnel: [w397 w410] -> w384
              tunnel: [w398 w403] -> w383
              tunnel: w376 -> [w398 w399]
              tunnel: w379 -> [_ w401]
              tunnel: w379 -> [_ w400]
              frame False {
              }
              frame True {
                n190 = call <vilib>:"GoTo.vi"("error in"=w399, "control refs"=w400) -> ("error out"=w409:errorcluster, "VisibleValue"=w406:u64)  [unwired: 8 in]
                n191 = property on="Temp Configuration" class="Clust (strict)"(error in=w409) -> (error out=w415:errorcluster, "Value"=w416:T1)  [unwired: 1 in, 1 out]
                n192 = call <vilib>:"UpdateBufferForMultiListBoxIfNecessary.vi"("control refs"=w401, "error in"=w415, "Buffer Configuration"=w416, "TDMS File Viewer Configuration"=w412, "tdms file in"=w411) -> ("error out"=w414:errorcluster, "BufferConfig out"=w413:T1, "tdms file out"=w410:refnum<k34>)  [unwired: 4 in]
                n193 = property on="Temp Configuration" class="Clust (strict)"(error in=w414, "Value"=w413) -> (error out=w402:errorcluster)  [unwired: 1 in, 1 out]
                n194 = property on="Raw data values" class="MCListbox (strict)"(error in=w402) -> (error out=w404:errorcluster, "TopLeft"=w408:T9)  [unwired: 1 in, 1 out]
                n195 = Unbundle By Name(w408) -> ("Row"=w407:u32)
                n196 = Add(x=w407, y=w406) -> (x+y=w405:u64)
                n197 = property on="Raw data values" class="MCListbox (strict)"(error in=w404, "Value"=w405) -> (error out=w403:errorcluster)  [unwired: 1 in, 1 out]
              }
            }
          }
          event Key Down? {
            n198 = event-data() -> ("VKey"=w421:T11)  [unwired: 1 out]
            n199 = case shown="\"F1\"" w421 {
              tunnel: [FALSE ("Discard?") TRUE ("Discard?")] -> w420
              frame Default {
              }
              frame "F1" {
                n200 = call <vilib>:"TDMSFileViewer_LaunchHelp.vi"("CHM or HLP filename (lvdialog.chm)"="lvdialog.chm", "HTML filename"="tdms_file_viewer_db.html") -> ()  [unwired: 1 in, 5 out]
              }
            }
            n201 = event-data("Discard?"=w420) -> ()  [unwired: 1 in, 1 out]
          }
          event "Waveform Graph": Shortcut Menu Selection (App) {
            n202 = event-data() -> ("ItemTag"=w432:string)  [unwired: 1 out]
            n203 = property on="Waveform Graph" class="WFGraph (strict)"(error in=w434) -> (error out=w427:errorcluster, "IgnoreTimestamp"=w431:bool)  [unwired: 1 in, 1 out]
            n204 = Not(x=w431) -> (.not. x?=w428:bool)
            n205 = Equal?(x=w432, y="APP_SC_IGNORE_TIME_STAMP") -> (x = y?=w429:bool)
            n206 = And(x=w428, y=w429) -> (x .and. y?=w430:bool)
            n207 = case shown="True" w430 {
              tunnel: w427 -> [w437 w441]
              tunnel: [w437 w438] -> w426
              frame False {
              }
              frame True {
                n208 = property on="LastXScaleFormat" class="DigNum (strict)"(error in=w441) -> (error out=w440:errorcluster, "Value"=w439:u8)  [unwired: 1 in, 1 out]
                n209 = property on="Waveform Graph" class="WFGraph (strict)"(error in=w440, "XScale.Format"=w439) -> (error out=w438:errorcluster)  [unwired: 1 in, 1 out]
              }
            }
          }
        }
      }
    }
    frame Error {
      n210 = call <vilib>:"Simple Error Handler.vi"("error in (no error)"=w444) -> ("error out"=w443:errorcluster)  [unwired: 1 in, 7 out]
    }
  }
  n211 = property class="Tree (strict)"(reference=w17, "Value"="") -> ()  [unwired: 1 in, 2 out]
  n212 = TDMS Close(8:w59, 11:w60) -> (0:w24:errorcluster)  [unwired: 1 out]
  n213 = case shown="True" w25 {
    tunnel: w24 -> [w446 w448]
    tunnel: [w446 w447] -> w5
    frame False {
    }
    frame True {
      n214 = invoke class="VI" method="FP.Close"(error in=w448) -> (error out=w447:errorcluster)  [unwired: 2 in, 2 out]
    }
  }
  n215 = Merge Errors(w11, w5) -> (→"error out":errorcluster)
